vi "Control - Load Command.vi"(11 "Control Inputs":T1={"Engine Speed [RPM]"=0.0, "Engine Status"=enum."STALLED", "Load Control \nMode"=enum."High-Idle Governor", "dt(s)"=0.0, "Number of Cylinders"=0, "Engine Displacement [cc]"=0.0, "StoichAFR"=0.0, "Q.LHV Fuel [kJ/kg]"=0.0, "BattV PSU [V]"=0.0, "12V PSU [V]"=0.0, "5V PSU [V]"=0.0, "Pedal Position [%]"=0.0, "Oil Pressure [kPa]"=0.0, "Oil Temp [C]"=0.0, "Oil Level [%]"=0.0, "Engine Coolant Temp (ECT) [C]"=0.0, "Engine Coolant Pressure [kPa]"=0.0, "Rail Pressure [bar]"=0.0, "Fuel Pressure [kPa]"=0.0, "Fuel Temp [C]"=0.0, "Vacuum Pressure [kPa]"=0.0, "Throttle Position [%]"=0.0, "Cam1 Advance [CAD]"=0.0, "Cam2 Advance [CAD]"=0.0, "Cam3 Advance [CAD]"=0.0, "Cam4 Advance [CAD]"=0.0, "CA50 Control Output [CAD]"=[], "CA50 Control Output Valid"=[], "Intake Air Temp (IAT) [C]"=0.0, "Barometric Air Pressure [kPa]"=0.0, "Intake Air Rel. Humidity [%]"=0.0, "Mass Air Flow (MAF) [kg/hr]"=0.0, "Turbo Inlet Air Pressure [kPa]"=0.0, "Turbo Inlet Air Temp [C]"=0.0, "Turbo Outlet Air Pressure [kPa]"=0.0, "Turbo Outlet Air Temp [C]"=0.0, "CAC Outlet Pressure [kPa]"=0.0, "CAC Outlet Temp [C]"=0.0, "Intake Manifold Pressure (MAP) [kPa]"=0.0, "Intake Manifold Temp (MAT) [C]"=0.0, "Exhaust Manifold Pressure [kPa]"=0.0, "Exhaust Manifold Temp [C]"=0.0, "HighP EGR Cooler Outlet Pressure [kPa]"=0.0, "HighP EGR Cooler Outlet Temp [C]"=0.0, "HighP EGR Differential Pressure [kPa]"=0.0, "HighP EGR Valve Position [%]"=0.0, "Turbo Outlet Exhaust Pressure [kPa]"=0.0, "Turbo Outlet Exhaust Temp [C]"=0.0, "VGT Position 1 [%]"=0.0, "VGT Position 2 [%]"=0.0, "Turbo Speed 1 [RPM]"=0.0, "Turbo Speed 2 [RPM]"=0.0, "LowP EGR Differential Pressure [kPa]"=0.0, "LowP EGR Valve Position [%]"=0.0, "UEGO1Lambda"=0.0, "UEGO1_Hot"=FALSE, "UEGO2Lambda"=0.0, "UEGO2_Hot"=FALSE, "Knock Intensity"=[], "Knock"=[]} {"Knock Intensity" format="%.2f"; "CA50 Control Output [CAD]" format="%.2f"; "Exhaust Manifold Temp [C]" format="%#_6f"; "UEGO2Lambda" format="%.2f"; "Intake Manifold Temp (MAT) [C]" format="%#_6f"; "UEGO1Lambda" format="%.2f"}) -> (0 "Pedal Desired [%]":sgl, 3 "MEP Desired [bar]":sgl)   [LabVIEW 2015, in "ECS-RT.lvlib"]
uses:
  ECS-RT.lvlib
  Typedefs/Control Inputs/Control Inputs.ctl
  Typedefs/EPT/Engine Status.ctl
  Typedefs/MISC/Load Control Mode.ctl
  ECS-Shared.lvlib
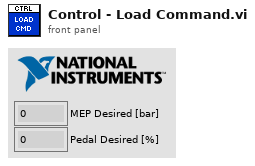
[diagram p1: front panel]
types:
  T1 = typedef "ECS-Shared.lvlib/Control Inputs.ctl" = cluster{"Engine Speed [RPM]":sgl, "Engine Status":T2, "Load Control \nMode":T3, "dt(s)":sgl, "Number of Cylinders":u8, "Engine Displacement [cc]":sgl, "StoichAFR":sgl, "Q.LHV Fuel [kJ/kg]":sgl, "BattV PSU [V]":sgl, "12V PSU [V]":sgl, "5V PSU [V]":sgl, "Pedal Position [%]":sgl, "Oil Pressure [kPa]":sgl, "Oil Temp [C]":sgl, "Oil Level [%]":sgl, "Engine Coolant Temp (ECT) [C]":sgl, "Engine Coolant Pressure [kPa]":sgl, "Rail Pressure [bar]":sgl, "Fuel Pressure [kPa]":sgl, "Fuel Temp [C]":sgl, "Vacuum Pressure [kPa]":sgl, "Throttle Position [%]":sgl, "Cam1 Advance [CAD]":sgl, "Cam2 Advance [CAD]":sgl, "Cam3 Advance [CAD]":sgl, "Cam4 Advance [CAD]":sgl, "CA50 Control Output [CAD]":sgl[], "CA50 Control Output Valid":bool[], "Intake Air Temp (IAT) [C]":sgl, "Barometric Air Pressure [kPa]":sgl, "Intake Air Rel. Humidity [%]":sgl, "Mass Air Flow (MAF) [kg/hr]":sgl, "Turbo Inlet Air Pressure [kPa]":sgl, "Turbo Inlet Air Temp [C]":sgl, "Turbo Outlet Air Pressure [kPa]":sgl, "Turbo Outlet Air Temp [C]":sgl, "CAC Outlet Pressure [kPa]":sgl, "CAC Outlet Temp [C]":sgl, "Intake Manifold Pressure (MAP) [kPa]":sgl, "Intake Manifold Temp (MAT) [C]":sgl, "Exhaust Manifold Pressure [kPa]":sgl, "Exhaust Manifold Temp [C]":sgl, "HighP EGR Cooler Outlet Pressure [kPa]":sgl, "HighP EGR Cooler Outlet Temp [C]":sgl, "HighP EGR Differential Pressure [kPa]":sgl, "HighP EGR Valve Position [%]":sgl, "Turbo Outlet Exhaust Pressure [kPa]":sgl, "Turbo Outlet Exhaust Temp [C]":sgl, "VGT Position 1 [%]":sgl, "VGT Position 2 [%]":sgl, "Turbo Speed 1 [RPM]":sgl, "Turbo Speed 2 [RPM]":sgl, "LowP EGR Differential Pressure [kPa]":sgl, "LowP EGR Valve Position [%]":sgl, "UEGO1Lambda":sgl, "UEGO1_Hot":bool, "UEGO2Lambda":sgl, "UEGO2_Hot":bool, "Knock Intensity":sgl[], "Knock":bool[]}
  T2 = typedef "ECS-Shared.lvlib/Engine Status.ctl" = enum16{"OFF", "STALLED", "CRANKING", "RUNNING", "ACCEL", "DECEL", "SAFE"}
  T3 = typedef "ECS-Shared.lvlib/Load Control Mode.ctl" = enum16{"No Governor", "Low-Idle Governor", "High-Idle Governor"}
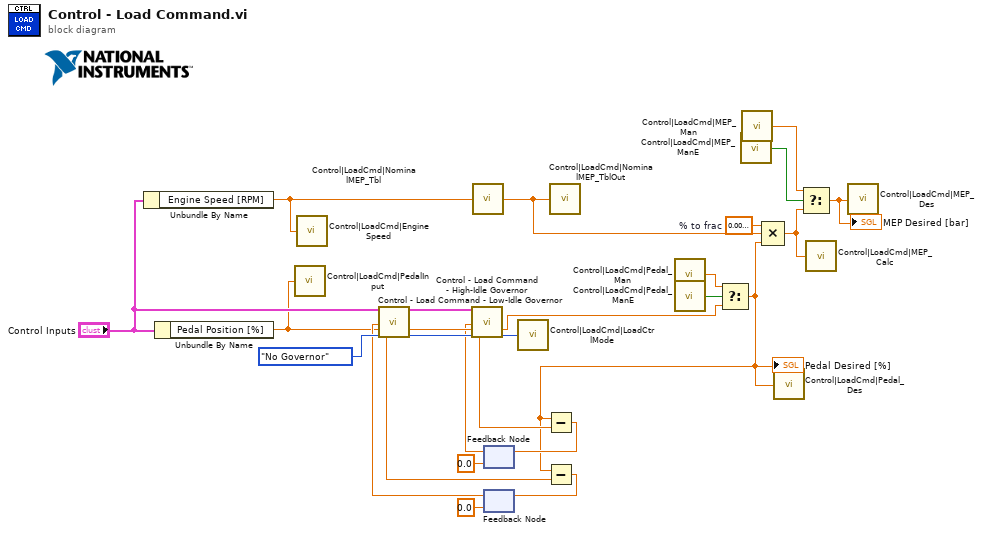
[diagram p0: block diagram]
diagram:
  w5 = sgl 0.01  # % to frac
  n1 = Unbundle By Name("Control Inputs") -> ("Engine Speed [RPM]"=w6:sgl)
  n2 = Unbundle By Name("Control Inputs") -> ("Pedal Position [%]"=w9:sgl)
  n3 = call "Control|LoadCmd|PedalInput"("Value"=w9) -> ()
  n4 = call "Control|LoadCmd|EngineSpeed"("Value"=w6) -> ()
  n5 = call "Control|LoadCmd|NominalMEP_Tbl"("X Index"=w6) -> ("Y"=w26:sgl)
  n6 = feedback #1(sgl 0.0) -> (w17:sgl)
  n7 = feedback #2(sgl 0.0) -> (w15:sgl)
  n8 = call "Control - Load Command - Low-Idle Governor.vi"("Control Inputs"="Control Inputs", "BeatbackDiff"=w15, "Pedal In"=w9, "Load Control Mode In"=Load_Control_Mode."No Governor") -> ("Governor Output"=w19:sgl, "Control Inputs"=w21:T1, "Pedal Out"=w24:sgl, "Load Control Mode Out"=w23:T3)  [unwired: 9 in, 3 out]
  n9 = call "Control - Load Command - High-Idle Governor.vi"("Control Inputs"=w21, "BeatbackDiff"=w17, "Pedal In"=w24, "Load Control Mode In"=w23) -> ("Governor Output"=w20:sgl, "Pedal Out"=w2:sgl, "Load Control Mode Out"=w12:T3)  [unwired: 9 in, 4 out]
  n10 = call "Control|LoadCmd|LoadCtrlMode"("Value"=w12) -> ()
  n11 = call "Control|LoadCmd|NominalMEP_TblOut"("Value"=w26) -> ()
  n12 = call "Control|LoadCmd|Pedal_Man"() -> ("Value"=w4:sgl)
  n13 = call "Control|LoadCmd|Pedal_ManE"() -> ("Value"=w3:bool)
  n14 = Select(t=w4, s=w3, f=w2) -> (s? t:f=w1:sgl)
  "Pedal Desired [%]" <- w1
  n15 = Subtract(x=w1, y=w20) -> (x-y=w18:sgl)
  n16 = feedback-in #1(w18) -> ()
  n17 = Subtract(x=w1, y=w19) -> (x-y=w16:sgl)
  n18 = feedback-in #2(w16) -> ()
  n19 = call "Control|LoadCmd|MEP_ManE"() -> ("Value"=w13:bool)
  n20 = call "Control|LoadCmd|MEP_Man"() -> ("Value"=w14:sgl)
  n21 = Compound Arithmetic op=MULTIPLY(w5, w26, w1) -> (w7:sgl)
  n22 = call "Control|LoadCmd|Pedal_Des"("Value"=w1) -> ()
  n23 = Select(t=w14, s=w13, f=w7) -> (s? t:f=w8:sgl)
  "MEP Desired [bar]" <- w8
  n24 = call "Control|LoadCmd|MEP_Calc"("Value"=w7) -> ()
  n25 = call "Control|LoadCmd|MEP_Des"("Value"=w8) -> ()
